vi "XPS_LTA_HS_Jogger.vi"(4 "Axis 2":string="Group7", 5 "Axis 1":string="Group2", 7 "Controller Address":string="192.168.254.254") -> ()   [LabVIEW 2016]
uses:
  <vilib>/Utility/miscctls.llb/LVMinMaxIncTypeDef.ctl
panel:
  in  "Data Entry Limits":T1
  in  "Axis Initial Parameters":T2={"Velocity (units/seconds)"=1.0, "Acceleration (units/seconds²)"=20.0, "Minimum Jerk Time (seconds)"=0.005, "Maximum Jerk Time (seconds)"=0.009} {"Maximum Jerk Time (seconds)" format="%.6e"; "Minimum Jerk Time (seconds)" format="%.6e"; "Acceleration (units/seconds²)" format="%.6e"; "Velocity (units/seconds)" format="%.6e"}
  in  "Mode selector":bool
  in  "Axis 2 Velocity (slow)\nmm/s":dbl=1.0 min=0.0 max=10.0 step=0.0001
  in  "Axis 2 Velocity (fast)\nmm/s":dbl=5.0 min=0.0 max=10.0 step=0.0001
  in  "Velocity (slow)":dbl=1.0 min=0.0 max=5.0 step=0.0001
  in  "Velocity (fast)":dbl=5.0 min=0.0 max=5.0 step=0.0001
  in  "Refresh Time":u32=100 min=50 max=10000 step=1
  in  "Tab Control":enum32{"JOG MODE", "MOVE MODE"}(tab)
  in  "Axis 1 negative":bool
  in  "Axis 1 negative fast":bool
  in  "Axis 1 Positive":bool
  in  "Axis 1 Positive fast":bool
  in  "Axis 2 negative":bool
  in  "Axis 2 negative fast":bool
  in  "Axis 2 Positive":bool
  in  "Axis 2 Positive fast":bool
  in  "Absolute":dbl=5.0 min=0.0 max=50.0
  in  "Absolute Axis 2":dbl=5.0 min=-75.0 max=75.0
  in  "Axis 1 move absolute":bool
  in  "Axis 2 move absolute":bool
  in  "Relative":dbl=1.0 min=-50.0 max=50.0
  in  "Relative Axis 2":dbl=1.0 min=-150.0 max=150.0
  in  "Axis 1 move relative":bool
  in  "Axis 2 move relative":bool
  out "Axis 1 Model":string
  out "Axis 2 Model":string
  in  "stop 2":bool
  out "Axis 2 position":dbl format="%.10f"
  out "Axis 2 Status":string
  out "Axis 1 position":dbl format="%.10f"
  out "Axis 1 Status":string
  in  "Motion parameter":T3={"Velocity (units/s)"=5.0, "Acceleration (units/s²)"=20.0} {"Acceleration (units/s²)" format="%.6f"; "Velocity (units/s)" format="%.6f"}
  in  "stop":bool
  # "Axis 1"
  # "Axis 2"
  # "msec"
  # "Axis 1"
  # "Axis 2"
  # "Axis 1"
  # "Axis 2"
  # "Absolute"
  # "Relative"
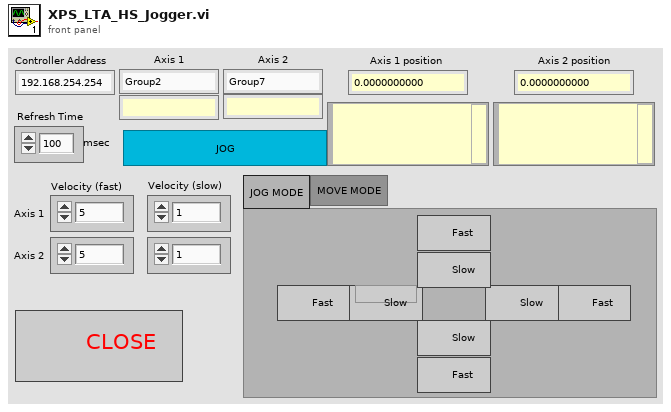
[diagram p1: front panel]
types:
  T1 = typedef "LVMinMaxIncTypeDef.ctl" = cluster{"Minimum":dbl, "Maximum":dbl, "Increment":dbl}
  T2 = cluster{"Velocity (units/seconds)":dbl, "Acceleration (units/seconds²)":dbl, "Minimum Jerk Time (seconds)":dbl, "Maximum Jerk Time (seconds)":dbl}
  T3 = cluster{"Velocity (units/s)":dbl, "Acceleration (units/s²)":dbl}
  T4 = enum32{"Page Enabled", "Page Disabled", "Page Disabled & Grayed"}
  T5 = cluster{"connection TCP":refnum<k5>, "LogTo File":bool, "Log File refnum":refnum<file>, "no error if error log":bool}
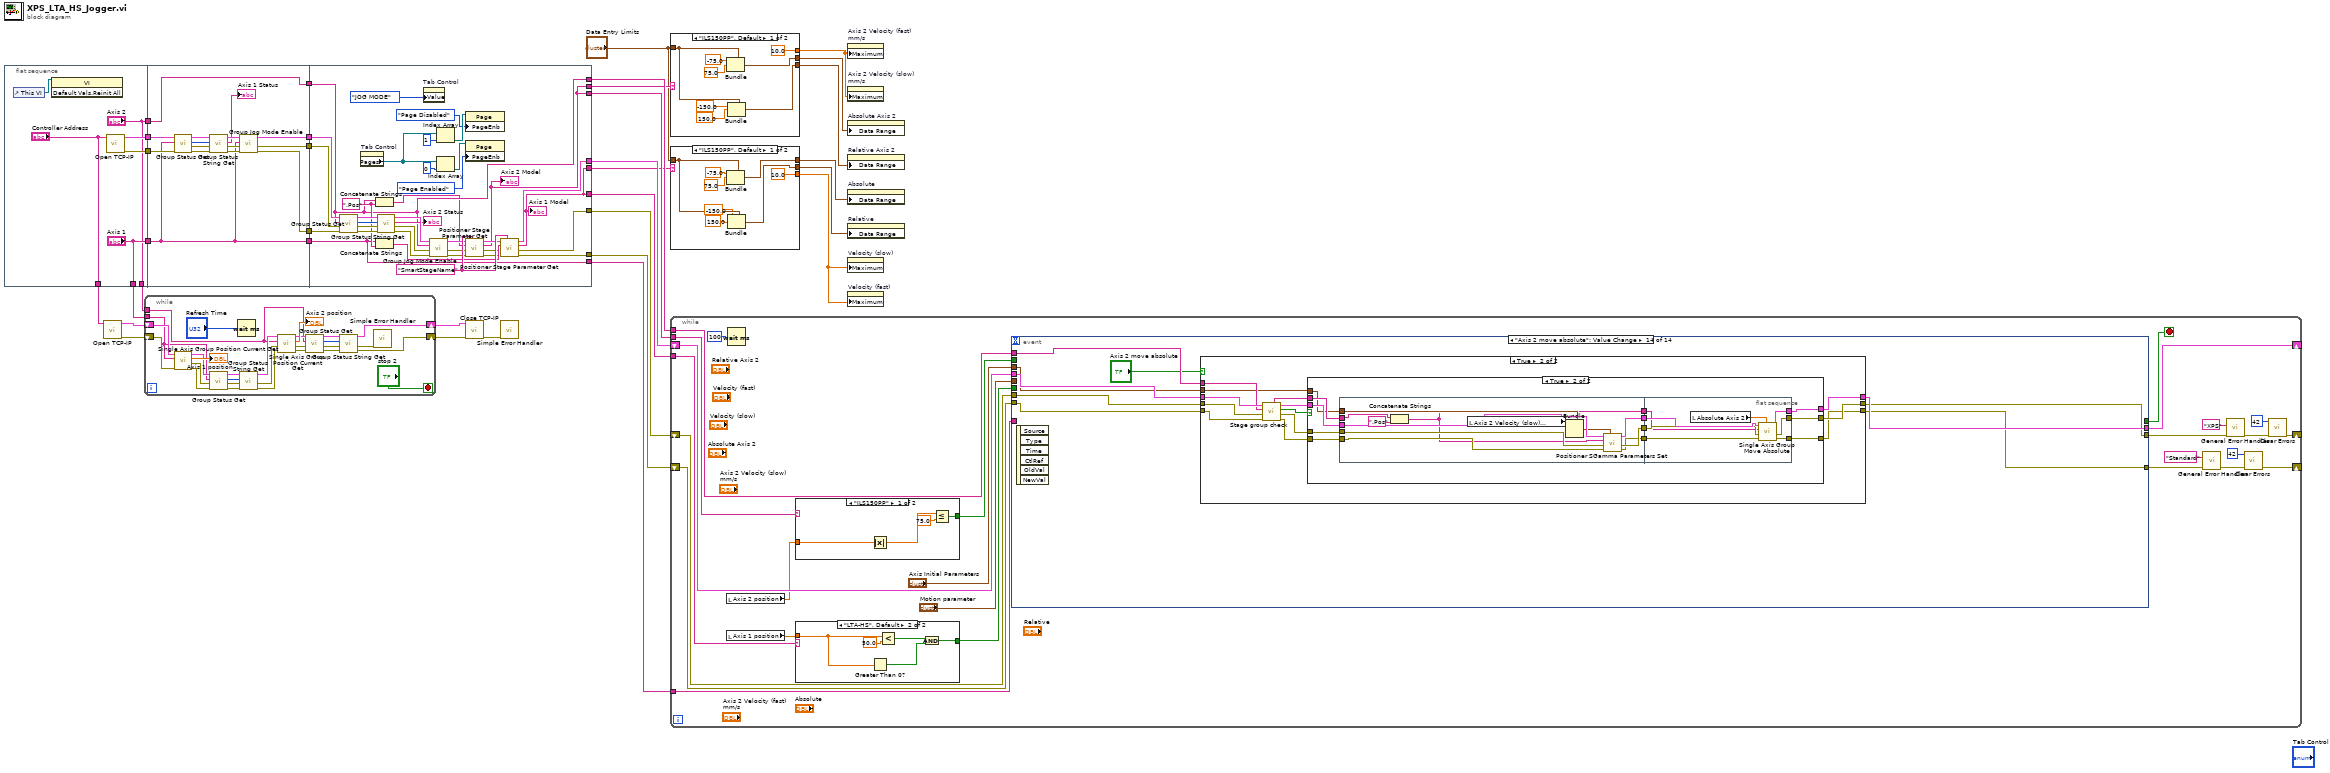
[diagram p0: block diagram]
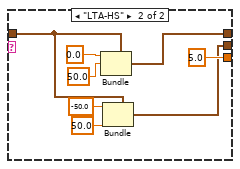
[diagram p2: hidden frame]
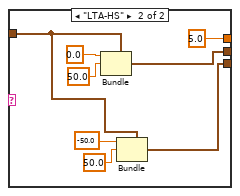
[diagram p3: hidden frame]
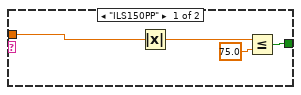
[diagram p4: hidden frame]
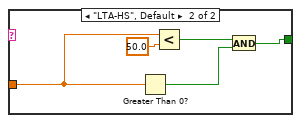
[diagram p5: hidden frame]
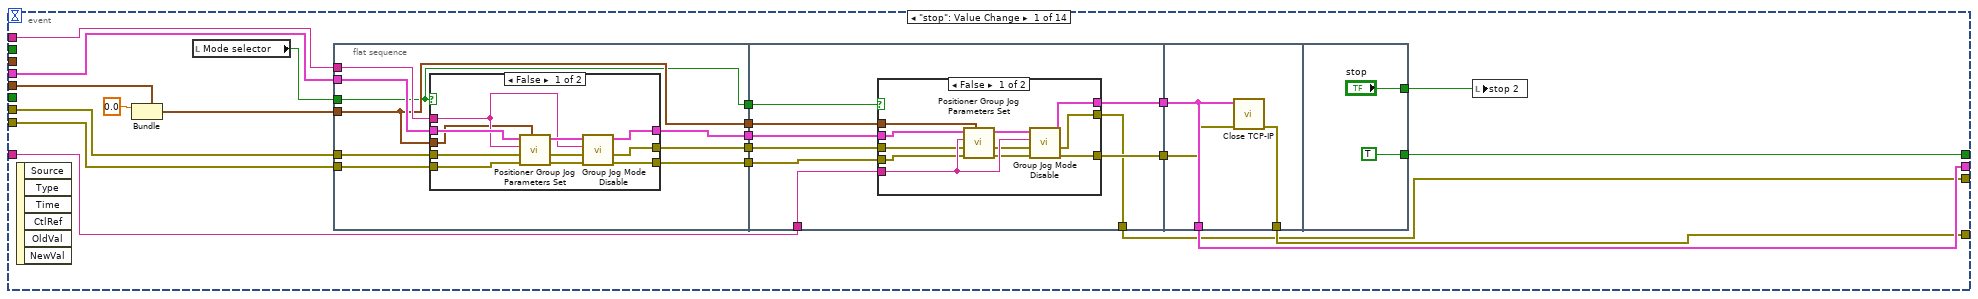
[diagram p6: hidden frame]
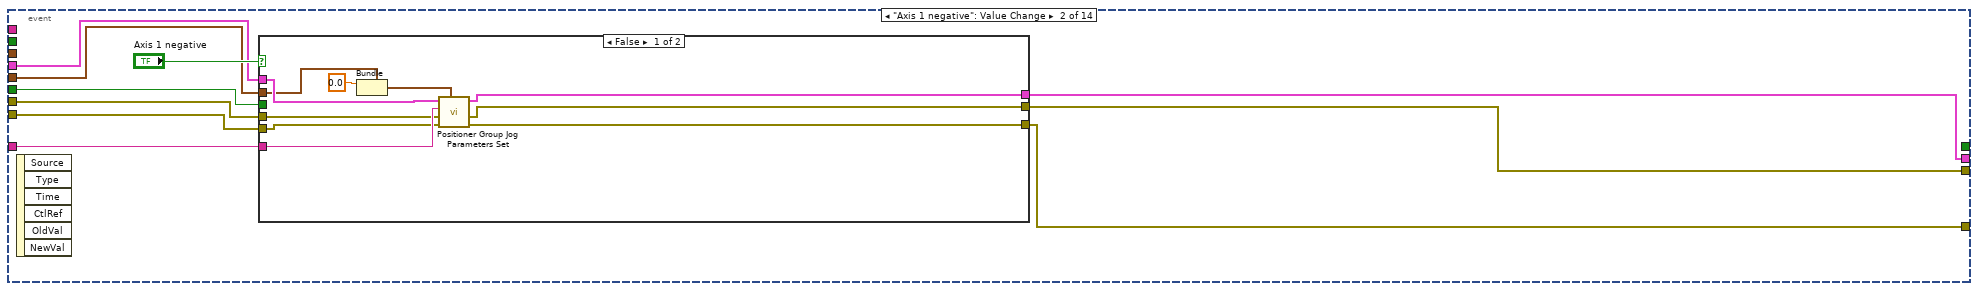
[diagram p9: hidden frame]
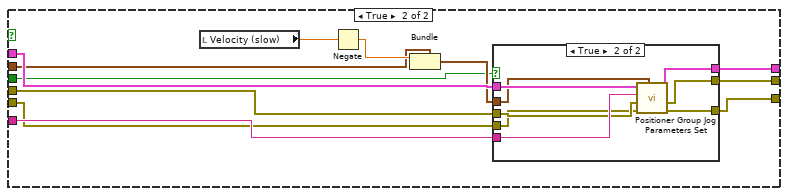
[diagram p10: hidden frame]
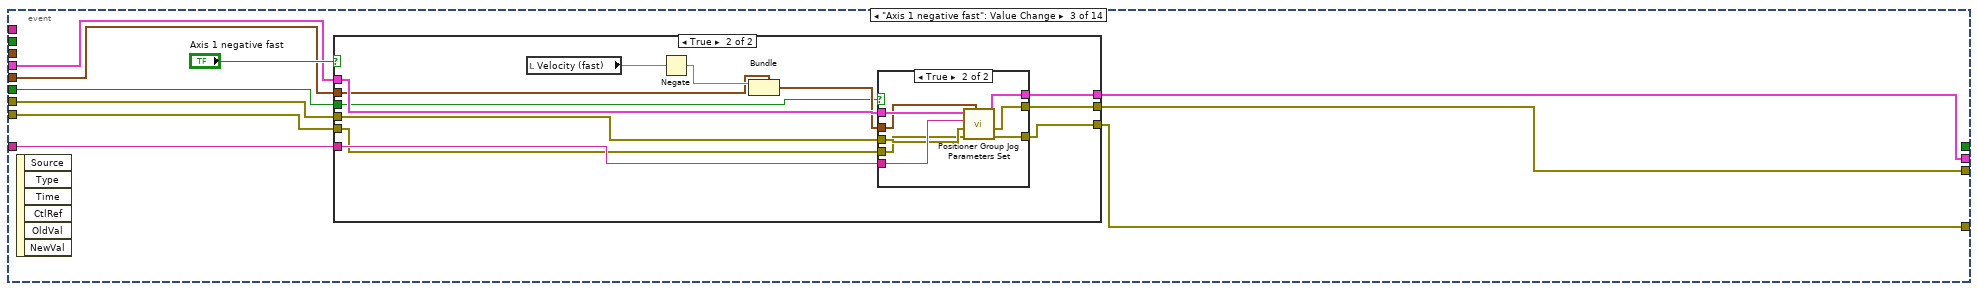
[diagram p12: hidden frame]
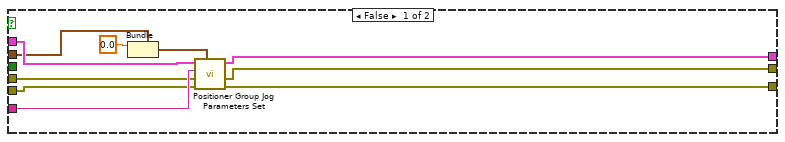
[diagram p13: hidden frame]
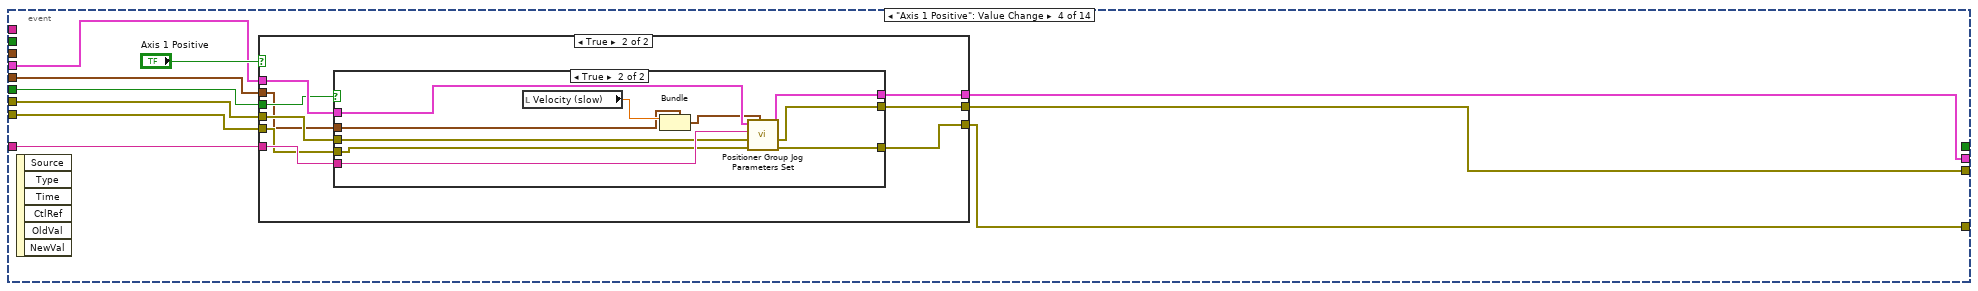
[diagram p15: hidden frame]
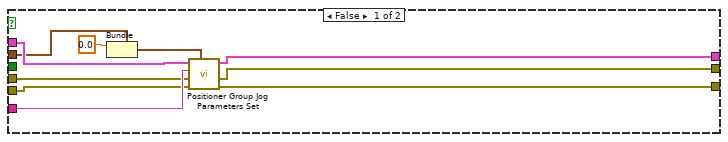
[diagram p16: hidden frame]
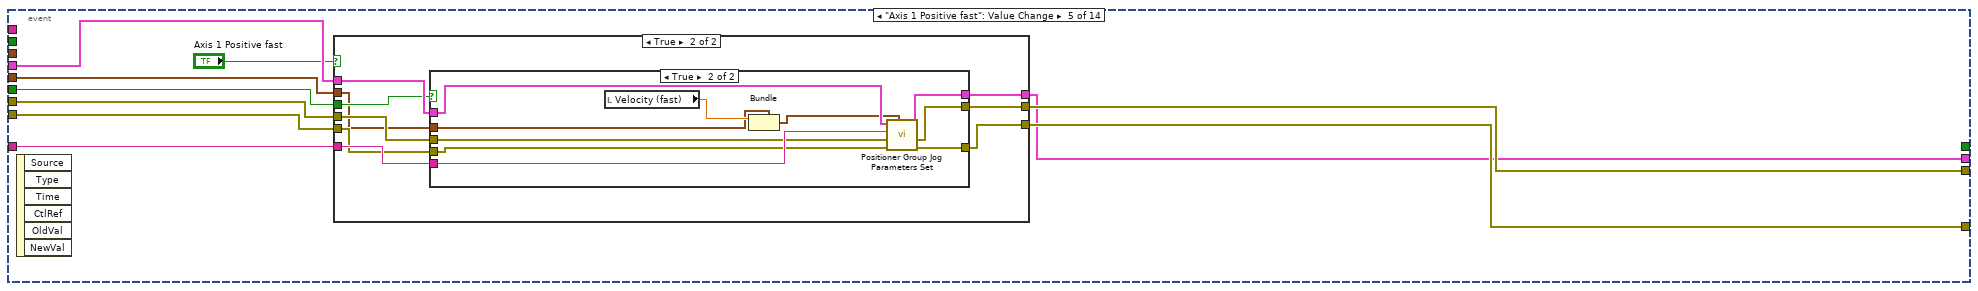
[diagram p18: hidden frame]
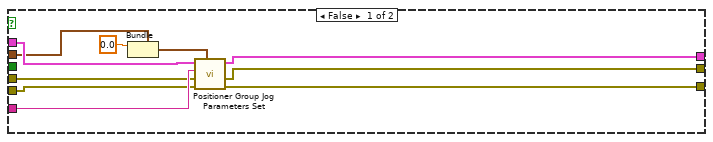
[diagram p19: hidden frame]
diagram:
  n1 = flat-sequence {
    tunnel: ["Axis 1"] -> w30
    tunnel: [w38] -> w29
    tunnel: [w37] -> w28
    tunnel: ["Axis 2"] -> w27
    tunnel: ["Controller Address"] -> w21
    tunnel: ["Axis 1"] -> w16
    tunnel: ["Axis 2"] -> w15
    tunnel: [w54] -> w33
    tunnel: [w53] -> w32
    tunnel: [w52] -> w31
    tunnel: w30 -> [w41]
    tunnel: w29 -> [w47]
    tunnel: w28 -> [w46]
    tunnel: w27 -> [w40]
    tunnel: [w40] -> w26
    tunnel: [w41] -> w24
    tunnel: w33 -> [w87]
    tunnel: w32 -> [w81]
    tunnel: w31 -> [w82]
    tunnel: w26 -> [w73]
    tunnel: w24 -> [w74]
    tunnel: [w65] -> w13
    tunnel: [w76] -> w25
    tunnel: [w74] -> w22
    tunnel: [w73] -> w23
    tunnel: [w68] -> w12
    tunnel: [w63] -> w11
    tunnel: [w64] -> w10
    tunnel: [w64] -> w9
    tunnel: [w63] -> w8
    frame #0 {
      n2 = control-ref of="This VI"() -> (w39:refnum<vi>)
      n3 = invoke class="VI" method="Default Vals.Reinit All"(reference=w39) -> ()  [unwired: 2 in, 3 out]
      n4 = call <userlib>:"Open TCP-IP.vi"("IP address"="Controller Address") -> ("error out"=w38:errorcluster, "Connection ID"=w37:T5)  [unwired: 5 in, 4 out]
    }
    frame #1 {
      n5 = call <userlib>:"Group Status Get.vi"("error in (no error)"=w47, "Group Name (250 c max)"=w41, "connection ID in"=w46) -> ("error out"=w50:errorcluster, "XPS error out"=w51:errorcluster, "Status"=w49:i32, "connection ID out"=w45:T5)  [unwired: 5 in]
      n6 = call <userlib>:"Group Status String Get.vi"("error in (no error)"=w50, "XPS error in (no error)"=w51, "Status #"=w49, "connection ID in"=w45) -> ("error out"=w44:errorcluster, "XPS error out"=w43:errorcluster, "Group Status String"=→"Axis 1 Status":string, "connection ID out"=w48:T5)  [unwired: 4 in]
      n7 = call <userlib>:"Group Jog Mode Enable.vi"("error in (no error)"=w44, "XPS error in (no error)"=w43, "Group Name (250 c max)"=w41, "connection ID in"=w48) -> ("error out"=w52:errorcluster, "XPS error out"=w53:errorcluster, "connection ID out"=w54:T5)  [unwired: 5 in]
    }
    frame #2 {
      w75 = ".Pos" ("string")
      w79 = "SmartStageName" ("Parameter Name (250 c max)")
      n8 = call <userlib>:"Group Status Get.vi"("error in (no error)"=w82, "XPS error in (no error)"=w81, "Group Name (250 c max)"=w73, "connection ID in"=w87) -> ("error out"=w89:errorcluster, "XPS error out"=w90:errorcluster, "Status"=w88:i32, "connection ID out"=w86:T5)  [unwired: 4 in]
      n9 = property on="Tab Control" class="TabCtl (strict)"() -> ("Pages"=w56:refnum<vi>[])  [unwired: 2 in, 2 out]
      n10 = Concatenate Strings(w73, w75) -> (w72:string)
      n11 = Concatenate Strings(w74, w75) -> (w71:string)
      n12 = call <userlib>:"Group Status String Get.vi"("error in (no error)"=w89, "XPS error in (no error)"=w90, "Status #"=w88, "connection ID in"=w86) -> ("error out"=w84:errorcluster, "XPS error out"=w83:errorcluster, "Group Status String"=→"Axis 2 Status":string, "connection ID out"=w85:T5)  [unwired: 4 in]
      n13 = property on="Tab Control" class="TabCtl (strict)"("Value"=enum32{"JOG MODE", "MOVE MODE"}."JOG MODE" ("Tab Control")) -> ()  [unwired: 2 in, 2 out]
      n14 = call <userlib>:"Group Jog Mode Enable.vi"("error in (no error)"=w84, "XPS error in (no error)"=w83, "Group Name (250 c max)"=w73, "connection ID in"=w85) -> ("error out"=w70:errorcluster, "XPS error out"=w67:errorcluster, "connection ID out"=w78:T5)  [unwired: 5 in]
      n15 = Index Array(array=w56, index=1) -> (element=w58:refnum<vi>)
      n16 = Index Array(array=w56, index=0) -> (element=w60:refnum<vi>)
      n17 = property class="Page"(reference=w58, "PageEnb"=T4."Page Disabled" ("Page Enabled State")) -> ()  [unwired: 1 in, 2 out]
      n18 = property class="Page"(reference=w60, "PageEnb"=T4."Page Enabled" ("Page Enabled State")) -> ()  [unwired: 1 in, 2 out]
      n19 = call <userlib>:"Positioner Stage Parameter Get.vi"("Parameter Name (250 c max)"=w79, "error in (no error)"=w70, "XPS error in (no error)"=w67, "Positioner Name (250 c max)"=w72, "connection ID in"=w78) -> ("error out"=w69:errorcluster, "XPS error out"=w66:errorcluster, "Parameter Value"=w64:string, "connection ID out"=w77:T5)  [unwired: 3 in]
      "Axis 2 Model" <- w64
      n20 = call <userlib>:"Positioner Stage Parameter Get.vi"("Parameter Name (250 c max)"=w79, "error in (no error)"=w69, "XPS error in (no error)"=w66, "Positioner Name (250 c max)"=w71, "connection ID in"=w77) -> ("error out"=w68:errorcluster, "XPS error out"=w65:errorcluster, "Parameter Value"=w63:string, "connection ID out"=w76:T5)  [unwired: 3 in]
      "Axis 1 Model" <- w63
    }
  }
  n21 = call <userlib>:"Open TCP-IP.vi"("IP address"=w21) -> ("error out"=w19:errorcluster, "Connection ID"=w20:T5)  [unwired: 5 in, 4 out]
  n22 = while {
    shift-right: [w93] -> w18
    shift-left: w20 -> [w118]
    shift-right: [w92] -> w17
    shift-left: w19 -> [w117]
    tunnel: w16 -> [w109]
    tunnel: w15 -> [w96]
    stop <- "stop 2" stop-if-true
    n23 = call <userlib>:"Single Axis Group Position Current Get.vi"("error in (no error)"=w117, "SingleAxis Group  Name (250 c max)"=w109, "connection ID in"=w118) -> ("error out"=w108:errorcluster, "XPS error out"=w107:errorcluster, "Current Position (units)"=→"Axis 1 position":dbl, "connection ID out"=w112:T5)  [unwired: 5 in]
    n24 = call <userlib>:"Group Status Get.vi"("error in (no error)"=w108, "XPS error in (no error)"=w107, "Group Name (250 c max)"=w109, "connection ID in"=w112) -> ("error out"=w105:errorcluster, "XPS error out"=w106:errorcluster, "Status"=w110:i32, "connection ID out"=w111:T5)  [unwired: 4 in]
    n25 = Wait (ms)(milliseconds to wait="Refresh Time") -> ()  [unwired: 1 out]
    n26 = call <userlib>:"Group Status String Get.vi"("error in (no error)"=w105, "XPS error in (no error)"=w106, "Status #"=w110, "connection ID in"=w111) -> ("error out"=w102:errorcluster, "XPS error out"=w103:errorcluster, "connection ID out"=w104:T5)  [unwired: 4 in, 1 out]
    n27 = call <userlib>:"Single Axis Group Position Current Get.vi"("error in (no error)"=w102, "XPS error in (no error)"=w103, "SingleAxis Group  Name (250 c max)"=w96, "connection ID in"=w104) -> ("error out"=w99:errorcluster, "XPS error out"=w100:errorcluster, "Current Position (units)"=→"Axis 2 position":dbl, "connection ID out"=w101:T5)  [unwired: 4 in]
    n28 = call <userlib>:"Group Status Get.vi"("error in (no error)"=w99, "XPS error in (no error)"=w100, "Group Name (250 c max)"=w96, "connection ID in"=w101) -> ("error out"=w97:errorcluster, "XPS error out"=w98:errorcluster, "Status"=w94:i32, "connection ID out"=w95:T5)  [unwired: 4 in]
    n29 = call <userlib>:"Group Status String Get.vi"("error in (no error)"=w97, "XPS error in (no error)"=w98, "Status #"=w94, "connection ID in"=w95) -> ("error out"=w92:errorcluster, "XPS error out"=w91:errorcluster, "connection ID out"=w93:T5)  [unwired: 4 in, 1 out]
    n30 = call <vilib>:"Simple Error Handler.vi"("error in (no error)"=w91) -> ()  [unwired: 4 in, 5 out]
  }
  n31 = call <userlib>:"Close TCP-IP.vi"("error in (no error)"=w17, "connection ID in"=w18) -> ("Error out"=w14:errorcluster)  [unwired: 9 in]
  n32 = call <vilib>:"Simple Error Handler.vi"("error in (no error)"=w14) -> ()  [unwired: 4 in, 5 out]
  n33 = case shown="\"ILS150PP\", Default" w9 {
    tunnel: [10.0 5.0] -> w7
    tunnel: "Data Entry Limits" -> [w122 w129]
    tunnel: [w123 w131] -> w4
    tunnel: [w120 w127] -> w3
    frame "ILS150PP", Default {
      n34 = Bundle(cluster=w122, "Minimum"=-75.0, "Maximum"=75.0) -> (w123:T1)  [unwired: 1 in]
      n35 = Bundle(cluster=w122, "Minimum"=-150.0, "Maximum"=150.0) -> (w120:T1)  [unwired: 1 in]
    }
    frame "LTA-HS" {
      n36 = Bundle(cluster=w129, "Minimum"=0.0, "Maximum"=50.0) -> (w131:T1)  [unwired: 1 in]
      n37 = Bundle(cluster=w129, "Minimum"=-50.0, "Maximum"=50.0) -> (w127:T1)  [unwired: 1 in]
    }
  }
  n38 = case shown="\"ILS150PP\", Default" w8 {
    tunnel: [10.0 5.0] -> w6
    tunnel: "Data Entry Limits" -> [w139 w146]
    tunnel: [w136 w143] -> w1
    tunnel: [w137 w147] -> w2
    frame "ILS150PP", Default {
      n39 = Bundle(cluster=w139, "Minimum"=-75.0, "Maximum"=75.0) -> (w137:T1)  [unwired: 1 in]
      n40 = Bundle(cluster=w139, "Minimum"=-150.0, "Maximum"=150.0) -> (w136:T1)  [unwired: 1 in]
    }
    frame "LTA-HS" {
      n41 = Bundle(cluster=w146, "Minimum"=0.0, "Maximum"=50.0) -> (w147:T1)  [unwired: 1 in]
      n42 = Bundle(cluster=w146, "Minimum"=-50.0, "Maximum"=50.0) -> (w143:T1)  [unwired: 1 in]
    }
  }
  n43 = while {
    shift-right: [w175] -> _
    shift-left: w25 -> [w176]
    tunnel: w23 -> [w174]
    tunnel: w22 -> [w173]
    shift-right: [w159] -> _
    shift-left: w12 -> [w166]
    shift-right: [w162] -> _
    shift-left: w13 -> [w167]
    tunnel: w11 -> [w154]
    tunnel: w10 -> [w153]
    stop <- w169 stop-if-true
    n44 = local read "Axis 2 position"() -> (w155:dbl)
    n45 = local read "Axis 1 position"() -> (w158:dbl)
    n46 = Wait (ms)(milliseconds to wait=u32 100) -> ()  [unwired: 1 out]
    n47 = case shown="\"ILS150PP\"" w153 {
      tunnel: w155 -> [w187 w192]
      tunnel: [w188 w190] -> w156
      frame "ILS150PP" {
        n48 = Absolute Value(x=w187) -> (abs(x)=w186:dbl)
        n49 = Less Or Equal?(x=w186, y=75.0) -> (x <= y?=w188:bool)
      }
      frame "LTA-HS", Default {
        n50 = Greater Than 0?(x=w192) -> (x > 0?=w191:bool)
        n51 = Less?(x=w192, y=50.0) -> (x < y?=w194:bool)
        n52 = And(x=w194, y=w191) -> (x .and. y?=w190:bool)
      }
    }
    n53 = case shown="\"LTA-HS\", Default" w154 {
      tunnel: w158 -> [w179 w183]
      tunnel: [w177 w181] -> w157
      frame "ILS150PP" {
        n54 = Absolute Value(x=w179) -> (abs(x)=w178:dbl)
        n55 = Less Or Equal?(x=w178, y=75.0) -> (x <= y?=w177:bool)
      }
      frame "LTA-HS", Default {
        n56 = Greater Than 0?(x=w183) -> (x > 0?=w182:bool)
        n57 = Less?(x=w183, y=50.0) -> (x < y?=w185:bool)
        n58 = And(x=w185, y=w182) -> (x .and. y?=w181:bool)
      }
    }
    n59 = event shown="[13] \"Axis 2 move absolute\": Value Change" {
      selector: _ -> [_ _ _ _ _ _ _ _ _ _ _ _ _ _]
      dyn-events: _ -> [_ _ _ _ _ _ _ _ _ _ _ _ _ _]
      timeout: _ -> [_ _ _ _ _ _ _ _ _ _ _ _ _ _]
      tunnel: [w200 w272 w315 w358 w403 w443 w485 w528 w570 w608 w773 w832 w893 w954] -> w170
      tunnel: w176 -> [w215 w275 w318 w361 w404 w445 w488 w531 w573 w615 w779 w839 w900 w962]
      tunnel: [w214 w274 w317 w360 w401 w442 w487 w530 w572 w610 w775 w834 w895 w956] -> w175
      tunnel: [w199 w273 w316 w359 w402 w444 w486 w529 w571 w609 w774 w833 w894 w955] -> w171
      tunnel: w174 -> [w209 _ _ _ _ w441 w484 w527 w569 w611 _ _ w898 w959]
      tunnel: w173 -> [w208 w271 w314 w357 w399 _ _ _ _ w614 w778 w836 _ _]
      tunnel: [w207 _ _ _ _ _ _ _ _ _ _ _ _ _] -> w169
      tunnel: w167 -> [w205 w270 w313 w356 w398 w440 w483 w526 w568 w613 w777 w838 w899 w961]
      tunnel: w166 -> [w201 w269 w312 w355 w397 w439 w482 w525 w567 w612 w776 w837 w897 w960]
      tunnel: w156 -> [_ _ _ _ _ w438 w481 w524 w566 _ _ _ _ _]
      tunnel: w157 -> [_ w268 w311 w354 w396 _ _ _ _ _ _ _ _ _]
      tunnel: "Axis Initial Parameters" -> [_ _ _ _ _ _ _ _ _ _ w772 w840 w901 w958]
      tunnel: "Motion parameter" -> [w198 w267 w310 w353 w395 w437 w480 w523 w565 w607 _ _ _ _]
      event "stop": Value Change {
        n60 = event-data() -> ()  [unwired: 1 in, 6 out]
        n61 = Bundle(cluster=w198, "Velocity (units/s)"=0.0) -> (w210:T3)  [unwired: 1 in]
        n62 = local read "Mode selector"() -> (w196:bool)
        n63 = flat-sequence {
          tunnel: w215 -> [w224]
          tunnel: [w223] -> w212
          tunnel: w210 -> [w217]
          tunnel: w209 -> [w222]
          tunnel: w205 -> [w221]
          tunnel: [w220] -> w204
          tunnel: [w219] -> w202
          tunnel: w201 -> [w218]
          tunnel: [w217] -> w197
          tunnel: w196 -> [w216]
          tunnel: [w216] -> w195
          tunnel: [w246] -> w213
          tunnel: w212 -> [w247]
          tunnel: w208 -> [w245]
          tunnel: w204 -> [w244]
          tunnel: [w243] -> w203
          tunnel: w202 -> [w242]
          tunnel: [w241] -> w199
          tunnel: w197 -> [w240]
          tunnel: w195 -> [w239]
          tunnel: [w264] -> w214
          tunnel: w213 -> [w264]
          tunnel: w203 -> [w263]
          tunnel: [w262] -> w200
          tunnel: [TRUE] -> w207
          tunnel: ["stop"] -> w206
          frame #0 {
            n64 = case shown="False" w216 {
              tunnel: w224 -> [w234 w238]
              tunnel: [w233 w238] -> w223
              tunnel: w222 -> [w232 _]
              tunnel: w221 -> [w231 w237]
              tunnel: [w229 w237] -> w220
              tunnel: [w228 w236] -> w219
              tunnel: w218 -> [w226 w236]
              tunnel: w217 -> [w225 _]
              frame False {
                n65 = call <userlib>:"Positioner Group Jog Parameters Set.vi"("Group Jog parameters"=w225, "error in (no error)"=w226, "XPS error in (no error)"=w231, "Positioner Name (250 c max)"=w232, "connection ID in"=w234) -> ("error out"=w227:errorcluster, "XPS error out"=w230:errorcluster, "connection ID out"=w235:T5)  [unwired: 4 in]
                n66 = call <userlib>:"Group Jog Mode Disable.vi"("error in (no error)"=w227, "XPS error in (no error)"=w230, "Group Name (250 c max)"=w232, "connection ID in"=w235) -> ("error out"=w228:errorcluster, "XPS error out"=w229:errorcluster, "connection ID out"=w233:T5)  [unwired: 5 in]
              }
              frame True {
              }
            }
          }
          frame #1 {
            n67 = case shown="False" w239 {
              tunnel: w247 -> [w258 w261]
              tunnel: [w256 w261] -> w246
              tunnel: w245 -> [w255 _]
              tunnel: w244 -> [w254 w260]
              tunnel: [w252 w259] -> w243
              tunnel: w242 -> [w250 w259]
              tunnel: [w249 w260] -> w241
              tunnel: w240 -> [w248 _]
              frame False {
                n68 = call <userlib>:"Positioner Group Jog Parameters Set.vi"("Group Jog parameters"=w248, "error in (no error)"=w250, "XPS error in (no error)"=w254, "Positioner Name (250 c max)"=w255, "connection ID in"=w258) -> ("error out"=w251:errorcluster, "XPS error out"=w253:errorcluster, "connection ID out"=w257:T5)  [unwired: 4 in]
                n69 = call <userlib>:"Group Jog Mode Disable.vi"("error in (no error)"=w251, "XPS error in (no error)"=w253, "Group Name (250 c max)"=w255, "connection ID in"=w257) -> ("error out"=w252:errorcluster, "XPS error out"=w249:errorcluster, "connection ID out"=w256:T5)  [unwired: 5 in]
              }
              frame True {
              }
            }
          }
          frame #2 {
            n70 = call <userlib>:"Close TCP-IP.vi"("error in (no error)"=w263, "connection ID in"=w264) -> ("Error out"=w262:errorcluster)  [unwired: 9 in]
          }
          frame #3 {
          }
        }
        n71 = local write "stop 2"(w206) -> ()
      }
      event "Axis 1 negative": Value Change {
        n72 = event-data() -> ()  [unwired: 1 in, 6 out]
        n73 = case shown="False" "Axis 1 negative" {
          tunnel: w275 -> [w286 w298]
          tunnel: [w285 w297] -> w274
          tunnel: [w284 w296] -> w273
          tunnel: [w283 w295] -> w272
          tunnel: w271 -> [w282 w294]
          tunnel: w270 -> [w280 w292]
          tunnel: w269 -> [w279 w291]
          tunnel: w268 -> [_ w290]
          tunnel: w267 -> [w278 w287]
          frame False {
            n74 = Bundle(cluster=w278, "Velocity (units/s)"=0.0) -> (w277:T3)  [unwired: 1 in]
            n75 = call <userlib>:"Positioner Group Jog Parameters Set.vi"("Group Jog parameters"=w277, "error in (no error)"=w279, "XPS error in (no error)"=w280, "Positioner Name (250 c max)"=w282, "connection ID in"=w286) -> ("error out"=w283:errorcluster, "XPS error out"=w284:errorcluster, "connection ID out"=w285:T5)  [unwired: 4 in]
          }
          frame True {
            n76 = local read "Velocity (slow)"() -> (w289:dbl)
            n77 = Negate(x=w289) -> (-x=w288:dbl)
            n78 = Bundle(cluster=w287, "Velocity (units/s)"=w288) -> (w293:T3)  [unwired: 1 in]
            n79 = case shown="True" w290 {
              tunnel: w298 -> [w301 w309]
              tunnel: [w301 w308] -> w297
              tunnel: [w300 w307] -> w296
              tunnel: [w299 w306] -> w295
              tunnel: w294 -> [_ w305]
              tunnel: w293 -> [_ w304]
              tunnel: w292 -> [w300 w303]
              tunnel: w291 -> [w299 w302]
              frame False {
              }
              frame True {
                n80 = call <userlib>:"Positioner Group Jog Parameters Set.vi"("Group Jog parameters"=w304, "error in (no error)"=w302, "XPS error in (no error)"=w303, "Positioner Name (250 c max)"=w305, "connection ID in"=w309) -> ("error out"=w306:errorcluster, "XPS error out"=w307:errorcluster, "connection ID out"=w308:T5)  [unwired: 4 in]
              }
            }
          }
        }
      }
      event "Axis 1 negative fast": Value Change {
        n81 = event-data() -> ()  [unwired: 1 in, 6 out]
        n82 = case shown="True" "Axis 1 negative fast" {
          tunnel: w318 -> [w329 w341]
          tunnel: [w328 w340] -> w317
          tunnel: [w327 w339] -> w316
          tunnel: [w326 w338] -> w315
          tunnel: w314 -> [w325 w337]
          tunnel: w313 -> [w323 w334]
          tunnel: w312 -> [w322 w333]
          tunnel: w311 -> [_ w332]
          tunnel: w310 -> [w321 w330]
          frame False {
            n83 = Bundle(cluster=w321, "Velocity (units/s)"=0.0) -> (w320:T3)  [unwired: 1 in]
            n84 = call <userlib>:"Positioner Group Jog Parameters Set.vi"("Group Jog parameters"=w320, "error in (no error)"=w322, "XPS error in (no error)"=w323, "Positioner Name (250 c max)"=w325, "connection ID in"=w329) -> ("error out"=w326:errorcluster, "XPS error out"=w327:errorcluster, "connection ID out"=w328:T5)  [unwired: 4 in]
          }
          frame True {
            n85 = local read "Velocity (fast)"() -> (w331:dbl)
            n86 = Negate(x=w331) -> (-x=w336:dbl)
            n87 = Bundle(cluster=w330, "Velocity (units/s)"=w336) -> (w335:T3)  [unwired: 1 in]
            n88 = case shown="True" w332 {
              tunnel: w341 -> [w342 w352]
              tunnel: [w342 w351] -> w340
              tunnel: [w343 w350] -> w339
              tunnel: [w344 w349] -> w338
              tunnel: w337 -> [_ w348]
              tunnel: w335 -> [_ w347]
              tunnel: w334 -> [w343 w346]
              tunnel: w333 -> [w344 w345]
              frame False {
              }
              frame True {
                n89 = call <userlib>:"Positioner Group Jog Parameters Set.vi"("Group Jog parameters"=w347, "error in (no error)"=w345, "XPS error in (no error)"=w346, "Positioner Name (250 c max)"=w348, "connection ID in"=w352) -> ("error out"=w349:errorcluster, "XPS error out"=w350:errorcluster, "connection ID out"=w351:T5)  [unwired: 4 in]
              }
            }
          }
        }
      }
      event "Axis 1 Positive": Value Change {
        n90 = event-data() -> ()  [unwired: 1 in, 6 out]
        n91 = case shown="True" "Axis 1 Positive" {
          tunnel: w361 -> [w372 w381]
          tunnel: [w371 w380] -> w360
          tunnel: [w370 w379] -> w359
          tunnel: [w369 w378] -> w358
          tunnel: w357 -> [w368 w377]
          tunnel: w356 -> [w366 w376]
          tunnel: w355 -> [w365 w375]
          tunnel: w354 -> [_ w374]
          tunnel: w353 -> [w364 w373]
          frame False {
            n92 = Bundle(cluster=w364, "Velocity (units/s)"=0.0) -> (w363:T3)  [unwired: 1 in]
            n93 = call <userlib>:"Positioner Group Jog Parameters Set.vi"("Group Jog parameters"=w363, "error in (no error)"=w365, "XPS error in (no error)"=w366, "Positioner Name (250 c max)"=w368, "connection ID in"=w372) -> ("error out"=w369:errorcluster, "XPS error out"=w370:errorcluster, "connection ID out"=w371:T5)  [unwired: 4 in]
          }
          frame True {
            n94 = case shown="True" w374 {
              tunnel: w381 -> [w382 w394]
              tunnel: [w382 w393] -> w380
              tunnel: [w384 w392] -> w379
              tunnel: [w383 w391] -> w378
              tunnel: w377 -> [_ w390]
              tunnel: w376 -> [w384 w389]
              tunnel: w375 -> [w383 w388]
              tunnel: w373 -> [_ w385]
              frame False {
              }
              frame True {
                n95 = local read "Velocity (slow)"() -> (w387:dbl)
                n96 = Bundle(cluster=w385, "Velocity (units/s)"=w387) -> (w386:T3)  [unwired: 1 in]
                n97 = call <userlib>:"Positioner Group Jog Parameters Set.vi"("Group Jog parameters"=w386, "error in (no error)"=w388, "XPS error in (no error)"=w389, "Positioner Name (250 c max)"=w390, "connection ID in"=w394) -> ("error out"=w391:errorcluster, "XPS error out"=w392:errorcluster, "connection ID out"=w393:T5)  [unwired: 4 in]
              }
            }
          }
        }
      }
      event "Axis 1 Positive fast": Value Change {
        n98 = event-data() -> ()  [unwired: 1 in, 6 out]
        n99 = case shown="True" "Axis 1 Positive fast" {
          tunnel: w404 -> [w414 w423]
          tunnel: [w411 w420] -> w403
          tunnel: [w412 w421] -> w402
          tunnel: [w413 w422] -> w401
          tunnel: w399 -> [w410 w419]
          tunnel: w398 -> [w408 w417]
          tunnel: w397 -> [w407 w418]
          tunnel: w396 -> [_ w416]
          tunnel: w395 -> [w406 w415]
          frame False {
            n100 = Bundle(cluster=w406, "Velocity (units/s)"=0.0) -> (w405:T3)  [unwired: 1 in]
            n101 = call <userlib>:"Positioner Group Jog Parameters Set.vi"("Group Jog parameters"=w405, "error in (no error)"=w407, "XPS error in (no error)"=w408, "Positioner Name (250 c max)"=w410, "connection ID in"=w414) -> ("error out"=w411:errorcluster, "XPS error out"=w412:errorcluster, "connection ID out"=w413:T5)  [unwired: 4 in]
          }
          frame True {
            n102 = case shown="True" w416 {
              tunnel: w423 -> [w424 w436]
              tunnel: [w424 w435] -> w422
              tunnel: [w426 w434] -> w421
              tunnel: [w425 w433] -> w420
              tunnel: w419 -> [_ w432]
              tunnel: w418 -> [w425 w431]
              tunnel: w417 -> [w426 w430]
              tunnel: w415 -> [_ w427]
              frame False {
              }
              frame True {
                n103 = local read "Velocity (fast)"() -> (w428:dbl)
                n104 = Bundle(cluster=w427, "Velocity (units/s)"=w428) -> (w429:T3)  [unwired: 1 in]
                n105 = call <userlib>:"Positioner Group Jog Parameters Set.vi"("Group Jog parameters"=w429, "error in (no error)"=w431, "XPS error in (no error)"=w430, "Positioner Name (250 c max)"=w432, "connection ID in"=w436) -> ("error out"=w433:errorcluster, "XPS error out"=w434:errorcluster, "connection ID out"=w435:T5)  [unwired: 4 in]
              }
            }
          }
        }
      }
      event "Axis 2 negative": Value Change {
        n106 = event-data() -> ()  [unwired: 1 in, 6 out]
        n107 = case shown="True" "Axis 2 negative" {
          tunnel: w445 -> [w456 w468]
          tunnel: [w454 w466] -> w444
          tunnel: [w453 w465] -> w443
          tunnel: [w455 w467] -> w442
          tunnel: w441 -> [w452 w464]
          tunnel: w440 -> [w450 w461]
          tunnel: w439 -> [w449 w460]
          tunnel: w438 -> [_ w459]
          tunnel: w437 -> [w448 w457]
          frame False {
            n108 = Bundle(cluster=w448, "Velocity (units/s)"=0.0) -> (w447:T3)  [unwired: 1 in]
            n109 = call <userlib>:"Positioner Group Jog Parameters Set.vi"("Group Jog parameters"=w447, "error in (no error)"=w449, "XPS error in (no error)"=w450, "Positioner Name (250 c max)"=w452, "connection ID in"=w456) -> ("error out"=w453:errorcluster, "XPS error out"=w454:errorcluster, "connection ID out"=w455:T5)  [unwired: 4 in]
          }
          frame True {
            n110 = local read "Axis 2 Velocity (slow)\nmm/s"() -> (w458:dbl)
            n111 = Negate(x=w458) -> (-x=w463:dbl)
            n112 = Bundle(cluster=w457, "Velocity (units/s)"=w463) -> (w462:T3)  [unwired: 1 in]
            n113 = case shown="True" w459 {
              tunnel: w468 -> [w471 w479]
              tunnel: [w471 w478] -> w467
              tunnel: [w470 w477] -> w466
              tunnel: [w469 w476] -> w465
              tunnel: w464 -> [_ w475]
              tunnel: w462 -> [_ w474]
              tunnel: w461 -> [w470 w473]
              tunnel: w460 -> [w469 w472]
              frame False {
              }
              frame True {
                n114 = call <userlib>:"Positioner Group Jog Parameters Set.vi"("Group Jog parameters"=w474, "error in (no error)"=w472, "XPS error in (no error)"=w473, "Positioner Name (250 c max)"=w475, "connection ID in"=w479) -> ("error out"=w476:errorcluster, "XPS error out"=w477:errorcluster, "connection ID out"=w478:T5)  [unwired: 4 in]
              }
            }
          }
        }
      }
      event "Axis 2 negative fast": Value Change {
        n115 = event-data() -> ()  [unwired: 1 in, 6 out]
        n116 = case shown="True" "Axis 2 negative fast" {
          tunnel: w488 -> [w499 w511]
          tunnel: [w498 w510] -> w487
          tunnel: [w497 w509] -> w486
          tunnel: [w496 w508] -> w485
          tunnel: w484 -> [w495 w507]
          tunnel: w483 -> [w493 w504]
          tunnel: w482 -> [w492 w503]
          tunnel: w481 -> [_ w502]
          tunnel: w480 -> [w491 w500]
          frame False {
            n117 = Bundle(cluster=w491, "Velocity (units/s)"=0.0) -> (w490:T3)  [unwired: 1 in]
            n118 = call <userlib>:"Positioner Group Jog Parameters Set.vi"("Group Jog parameters"=w490, "error in (no error)"=w492, "XPS error in (no error)"=w493, "Positioner Name (250 c max)"=w495, "connection ID in"=w499) -> ("error out"=w496:errorcluster, "XPS error out"=w497:errorcluster, "connection ID out"=w498:T5)  [unwired: 4 in]
          }
          frame True {
            n119 = local read "Axis 2 Velocity (fast)\nmm/s"() -> (w501:dbl)
            n120 = Negate(x=w501) -> (-x=w506:dbl)
            n121 = Bundle(cluster=w500, "Velocity (units/s)"=w506) -> (w505:T3)  [unwired: 1 in]
            n122 = case shown="True" w502 {
              tunnel: w511 -> [w514 w522]
              tunnel: [w514 w521] -> w510
              tunnel: [w513 w520] -> w509
              tunnel: [w512 w519] -> w508
              tunnel: w507 -> [_ w518]
              tunnel: w505 -> [_ w517]
              tunnel: w504 -> [w513 w516]
              tunnel: w503 -> [w512 w515]
              frame False {
              }
              frame True {
                n123 = call <userlib>:"Positioner Group Jog Parameters Set.vi"("Group Jog parameters"=w517, "error in (no error)"=w515, "XPS error in (no error)"=w516, "Positioner Name (250 c max)"=w518, "connection ID in"=w522) -> ("error out"=w519:errorcluster, "XPS error out"=w520:errorcluster, "connection ID out"=w521:T5)  [unwired: 4 in]
              }
            }
          }
        }
      }
      event "Axis 2 Positive": Value Change {
        n124 = event-data() -> ()  [unwired: 1 in, 6 out]
        n125 = case shown="True" "Axis 2 Positive" {
          tunnel: w531 -> [w542 w551]
          tunnel: [w541 w550] -> w530
          tunnel: [w540 w549] -> w529
          tunnel: [w539 w548] -> w528
          tunnel: w527 -> [w538 w547]
          tunnel: w526 -> [w535 w546]
          tunnel: w525 -> [w536 w545]
          tunnel: w524 -> [_ w544]
          tunnel: w523 -> [w534 w543]
          frame False {
            n126 = Bundle(cluster=w534, "Velocity (units/s)"=0.0) -> (w533:T3)  [unwired: 1 in]
            n127 = call <userlib>:"Positioner Group Jog Parameters Set.vi"("Group Jog parameters"=w533, "error in (no error)"=w536, "XPS error in (no error)"=w535, "Positioner Name (250 c max)"=w538, "connection ID in"=w542) -> ("error out"=w539:errorcluster, "XPS error out"=w540:errorcluster, "connection ID out"=w541:T5)  [unwired: 4 in]
          }
          frame True {
            n128 = case shown="True" w544 {
              tunnel: w551 -> [w554 w564]
              tunnel: [w554 w563] -> w550
              tunnel: [w553 w562] -> w549
              tunnel: [w552 w561] -> w548
              tunnel: w547 -> [_ w560]
              tunnel: w546 -> [w553 w559]
              tunnel: w545 -> [w552 w558]
              tunnel: w543 -> [_ w555]
              frame False {
              }
              frame True {
                n129 = local read "Axis 2 Velocity (slow)\nmm/s"() -> (w556:dbl)
                n130 = Bundle(cluster=w555, "Velocity (units/s)"=w556) -> (w557:T3)  [unwired: 1 in]
                n131 = call <userlib>:"Positioner Group Jog Parameters Set.vi"("Group Jog parameters"=w557, "error in (no error)"=w558, "XPS error in (no error)"=w559, "Positioner Name (250 c max)"=w560, "connection ID in"=w564) -> ("error out"=w561:errorcluster, "XPS error out"=w562:errorcluster, "connection ID out"=w563:T5)  [unwired: 4 in]
              }
            }
          }
        }
      }
      event "Axis 2 Positive fast": Value Change {
        n132 = event-data() -> ()  [unwired: 1 in, 6 out]
        n133 = case shown="True" "Axis 2 Positive fast" {
          tunnel: w573 -> [w584 w593]
          tunnel: [w583 w590] -> w572
          tunnel: [w582 w591] -> w571
          tunnel: [w581 w592] -> w570
          tunnel: w569 -> [w580 w589]
          tunnel: w568 -> [w577 w588]
          tunnel: w567 -> [w578 w587]
          tunnel: w566 -> [_ w586]
          tunnel: w565 -> [w576 w585]
          frame False {
            n134 = Bundle(cluster=w576, "Velocity (units/s)"=0.0) -> (w575:T3)  [unwired: 1 in]
            n135 = call <userlib>:"Positioner Group Jog Parameters Set.vi"("Group Jog parameters"=w575, "error in (no error)"=w578, "XPS error in (no error)"=w577, "Positioner Name (250 c max)"=w580, "connection ID in"=w584) -> ("error out"=w581:errorcluster, "XPS error out"=w582:errorcluster, "connection ID out"=w583:T5)  [unwired: 4 in]
          }
          frame True {
            n136 = case shown="True" w586 {
              tunnel: w593 -> [w596 w606]
              tunnel: [w594 w605] -> w592
              tunnel: [w595 w604] -> w591
              tunnel: [w596 w603] -> w590
              tunnel: w589 -> [_ w602]
              tunnel: w588 -> [w595 w601]
              tunnel: w587 -> [w594 w600]
              tunnel: w585 -> [_ w597]
              frame False {
              }
              frame True {
                n137 = local read "Axis 2 Velocity (fast)\nmm/s"() -> (w598:dbl)
                n138 = Bundle(cluster=w597, "Velocity (units/s)"=w598) -> (w599:T3)  [unwired: 1 in]
                n139 = call <userlib>:"Positioner Group Jog Parameters Set.vi"("Group Jog parameters"=w599, "error in (no error)"=w600, "XPS error in (no error)"=w601, "Positioner Name (250 c max)"=w602, "connection ID in"=w606) -> ("error out"=w605:errorcluster, "XPS error out"=w604:errorcluster, "connection ID out"=w603:T5)  [unwired: 4 in]
              }
            }
          }
        }
      }
      event "Mode selector": Value Change {
        n140 = event-data() -> ()  [unwired: 1 in, 6 out]
        n141 = case shown="False" "Mode selector" {
          tunnel: w615 -> [w631 w701]
          tunnel: w614 -> [w627 w699]
          tunnel: w613 -> [w630 w697]
          tunnel: w612 -> [w629 w696]
          tunnel: w611 -> [w628 w698]
          tunnel: [w634 w712] -> w610
          tunnel: [w633 w711] -> w609
          tunnel: [w632 w710] -> w608
          tunnel: w607 -> [_ w695]
          frame False {
            n142 = call "Stage group check.vi"("error in (no error)"=w629, "XPS error in (no error)"=w630, "Group Name (250 c max)"=w627, "connection ID in"=w631) -> ("error out"=w619:errorcluster, "XPS error out"=w620:errorcluster, "Stages ready?"=w617:bool, "connection ID out"=w624:T5, "Group Name (250 c max) 2"=w626:string)  [unwired: 3 in]
            n143 = call "Stage group check.vi"("error in (no error)"=w619, "XPS error in (no error)"=w620, "Group Name (250 c max)"=w628, "connection ID in"=w624) -> ("error out"=w621:errorcluster, "XPS error out"=w622:errorcluster, "Stages ready?"=w618:bool, "connection ID out"=w623:T5, "Group Name (250 c max) 2"=w625:string)  [unwired: 3 in]
            n144 = And(x=w617, y=w618) -> (x .and. y?=w635:bool)
            n145 = case shown="True" w635 {
              tunnel: [w636 w651] -> w634
              tunnel: [w637 w650] -> w633
              tunnel: [w638 w649] -> w632
              tunnel: w625 -> [_ w647]
              tunnel: w626 -> [_ w646]
              tunnel: w623 -> [w636 w645]
              tunnel: w622 -> [w637 w644]
              tunnel: w621 -> [w638 w643]
              frame False {
                n146 = One Button Dialog(message="Axes are not ready") -> ()  [unwired: 1 in, 1 out]
              }
              frame True {
                n147 = flat-sequence {
                  tunnel: [w660] -> w653
                  tunnel: [w659] -> w652
                  tunnel: [w658] -> w648
                  tunnel: w646 -> [w657]
                  tunnel: w645 -> [w656]
                  tunnel: w644 -> [w655]
                  tunnel: w643 -> [w654]
                  tunnel: w653 -> [w675]
                  tunnel: w652 -> [w674]
                  tunnel: w648 -> [w670]
                  tunnel: w647 -> [w669]
                  tunnel: [w673] -> w642
                  tunnel: [w672] -> w641
                  tunnel: [w671] -> w640
                  tunnel: [w692] -> w649
                  tunnel: [w693] -> w650
                  tunnel: [w694] -> w651
                  tunnel: w642 -> [w694]
                  tunnel: w641 -> [w693]
                  tunnel: w640 -> [w692]
                  frame #0 {
                    n148 = call <userlib>:"Group Status Get.vi"("error in (no error)"=w654, "XPS error in (no error)"=w655, "Group Name (250 c max)"=w657, "connection ID in"=w656) -> ("error out"=w667:errorcluster, "XPS error out"=w668:errorcluster, "Status"=w666:i32, "connection ID out"=w664:T5)  [unwired: 4 in]
                    n149 = call <userlib>:"Group Status String Get.vi"("error in (no error)"=w667, "XPS error in (no error)"=w668, "Status #"=w666, "connection ID in"=w664) -> ("error out"=w663:errorcluster, "XPS error out"=w662:errorcluster, "Group Status String"=w661:string, "connection ID out"=w665:T5)  [unwired: 4 in]
                    n150 = local write "Axis 1 Status"(w661) -> ()
                    n151 = call <userlib>:"Group Jog Mode Enable.vi"("error in (no error)"=w663, "XPS error in (no error)"=w662, "Group Name (250 c max)"=w657, "connection ID in"=w665) -> ("error out"=w660:errorcluster, "XPS error out"=w659:errorcluster, "connection ID out"=w658:T5)  [unwired: 5 in]
                  }
                  frame #1 {
                    n152 = call <userlib>:"Group Status Get.vi"("error in (no error)"=w675, "XPS error in (no error)"=w674, "Group Name (250 c max)"=w669, "connection ID in"=w670) -> ("error out"=w682:errorcluster, "XPS error out"=w683:errorcluster, "Status"=w681:i32, "connection ID out"=w679:T5)  [unwired: 4 in]
                    n153 = call <userlib>:"Group Status String Get.vi"("error in (no error)"=w682, "XPS error in (no error)"=w683, "Status #"=w681, "connection ID in"=w679) -> ("error out"=w678:errorcluster, "XPS error out"=w677:errorcluster, "Group Status String"=w676:string, "connection ID out"=w680:T5)  [unwired: 4 in]
                    n154 = local write "Axis 2 Status"(w676) -> ()
                    n155 = call <userlib>:"Group Jog Mode Enable.vi"("error in (no error)"=w678, "XPS error in (no error)"=w677, "Group Name (250 c max)"=w669, "connection ID in"=w680) -> ("error out"=w671:errorcluster, "XPS error out"=w672:errorcluster, "connection ID out"=w673:T5)  [unwired: 5 in]
                  }
                  frame #2 {
                    n156 = property on="Tab Control" class="TabCtl (strict)"() -> ("Pages"=w685:refnum<vi>[])  [unwired: 2 in, 2 out]
                    n157 = property on="Tab Control" class="TabCtl (strict)"("Value"=enum32{"JOG MODE", "MOVE MODE"}."JOG MODE" ("Tab Control")) -> ()  [unwired: 2 in, 2 out]
                    n158 = Index Array(array=w685, index=1) -> (element=w687:refnum<vi>)
                    n159 = Index Array(array=w685, index=0) -> (element=w689:refnum<vi>)
                    n160 = property class="Page"(reference=w687, "PageEnb"=T4."Page Disabled" ("Page Enabled State")) -> ()  [unwired: 1 in, 2 out]
                    n161 = property class="Page"(reference=w689, "PageEnb"=T4."Page Enabled" ("Page Enabled State")) -> ()  [unwired: 1 in, 2 out]
                  }
                }
              }
            }
          }
          frame True {
            w704 = 44
            n162 = call <userlib>:"Group Status Get.vi"("error in (no error)"=w696, "XPS error in (no error)"=w697, "Group Name (250 c max)"=w698, "connection ID in"=w701) -> ("error out"=w708:errorcluster, "XPS error out"=w707:errorcluster, "Status"=w705:i32, "connection ID out"=w709:T5)  [unwired: 4 in]
            n163 = call <userlib>:"Group Status Get.vi"("error in (no error)"=w708, "XPS error in (no error)"=w707, "Group Name (250 c max)"=w699, "connection ID in"=w709) -> ("error out"=w702:errorcluster, "XPS error out"=w703:errorcluster, "Status"=w706:i32, "connection ID out"=w700:T5)  [unwired: 4 in]
            n164 = Equal?(x=w705, y=w704) -> (x = y?=w714:bool)
            n165 = Equal?(x=w706, y=w704) -> (x = y?=w715:bool)
            n166 = And(x=w715, y=w714) -> (x .and. y?=w713:bool)
            n167 = case shown="False" w713 {
              tunnel: w700 -> [w731 w767]
              tunnel: w699 -> [w730 _]
              tunnel: w703 -> [w729 w769]
              tunnel: w702 -> [w728 w768]
              tunnel: w698 -> [w724 _]
              tunnel: [w723 w767] -> w712
              tunnel: [w722 w769] -> w711
              tunnel: [w721 w768] -> w710
              tunnel: w695 -> [w717 _]
              frame False {
                n168 = flat-sequence {
                  tunnel: w731 -> [w740]
                  tunnel: w730 -> [w737]
                  tunnel: w729 -> [w739]
                  tunnel: w728 -> [w738]
                  tunnel: [w736] -> w727
                  tunnel: [w735] -> w726
                  tunnel: [w734] -> w725
                  tunnel: w717 -> [w733]
                  tunnel: [w732] -> w716
                  tunnel: w727 -> [w752]
                  tunnel: w726 -> [w751]
                  tunnel: w725 -> [w750]
                  tunnel: w724 -> [w749]
                  tunnel: [w748] -> w720
                  tunnel: [w747] -> w719
                  tunnel: [w746] -> w718
                  tunnel: w716 -> [w745]
                  tunnel: [w764] -> w721
                  tunnel: [w765] -> w722
                  tunnel: [w766] -> w723
                  tunnel: w720 -> [w766]
                  tunnel: w719 -> [w765]
                  tunnel: w718 -> [w764]
                  frame #0 {
                    n169 = Bundle(cluster=w733, "Velocity (units/s)"=0.0) -> (w732:T3)  [unwired: 1 in]
                    n170 = call <userlib>:"Positioner Group Jog Parameters Set.vi"("Group Jog parameters"=w732, "error in (no error)"=w738, "XPS error in (no error)"=w739, "Positioner Name (250 c max)"=w737, "connection ID in"=w740) -> ("error out"=w741:errorcluster, "XPS error out"=w742:errorcluster, "connection ID out"=w743:T5)  [unwired: 4 in]
                    n171 = call <userlib>:"Group Jog Mode Disable.vi"("error in (no error)"=w741, "XPS error in (no error)"=w742, "Group Name (250 c max)"=w737, "connection ID in"=w743) -> ("error out"=w734:errorcluster, "XPS error out"=w735:errorcluster, "connection ID out"=w736:T5)  [unwired: 5 in]
                  }
                  frame #1 {
                    n172 = call <userlib>:"Positioner Group Jog Parameters Set.vi"("Group Jog parameters"=w745, "error in (no error)"=w750, "XPS error in (no error)"=w751, "Positioner Name (250 c max)"=w749, "connection ID in"=w752) -> ("error out"=w755:errorcluster, "XPS error out"=w754:errorcluster, "connection ID out"=w753:T5)  [unwired: 4 in]
                    n173 = call <userlib>:"Group Jog Mode Disable.vi"("error in (no error)"=w755, "XPS error in (no error)"=w754, "Group Name (250 c max)"=w749, "connection ID in"=w753) -> ("error out"=w746:errorcluster, "XPS error out"=w747:errorcluster, "connection ID out"=w748:T5)  [unwired: 5 in]
                  }
                  frame #2 {
                    n174 = property on="Tab Control" class="TabCtl (strict)"() -> ("Pages"=w757:refnum<vi>[])  [unwired: 2 in, 2 out]
                    n175 = Index Array(array=w757, index=1) -> (element=w759:refnum<vi>)
                    n176 = Index Array(array=w757, index=0) -> (element=w761:refnum<vi>)
                    n177 = property on="Tab Control" class="TabCtl (strict)"("Value"=enum32{"JOG MODE", "MOVE MODE"}."MOVE MODE" ("Tab Control")) -> ()  [unwired: 2 in, 2 out]
                    n178 = property class="Page"(reference=w759, "PageEnb"=T4."Page Enabled" ("Page Enabled State")) -> ()  [unwired: 1 in, 2 out]
                    n179 = property class="Page"(reference=w761, "PageEnb"=T4."Page Disabled" ("Page Enabled State")) -> ()  [unwired: 1 in, 2 out]
                  }
                }
              }
              frame True {
                n180 = One Button Dialog(message="Axes are still moving") -> ()  [unwired: 1 in, 1 out]
              }
            }
          }
        }
      }
      event "Axis 1 move absolute": Value Change {
        n181 = event-data() -> ()  [unwired: 1 in, 6 out]
        n182 = case shown="True" "Axis 1 move absolute" {
          tunnel: w779 -> [w782 w794]
          tunnel: w778 -> [_ w793]
          tunnel: w777 -> [w781 w792]
          tunnel: w776 -> [w780 w791]
          tunnel: [w782 w789] -> w775
          tunnel: [w781 w787] -> w774
          tunnel: [w780 w785] -> w773
          tunnel: w772 -> [_ w783]
          frame False {
          }
          frame True {
            n183 = call "Stage group check.vi"("error in (no error)"=w791, "XPS error in (no error)"=w792, "Group Name (250 c max)"=w793, "connection ID in"=w794) -> ("error out"=w786:errorcluster, "XPS error out"=w788:errorcluster, "Stages ready?"=w795:bool, "connection ID out"=w790:T5, "Group Name (250 c max) 2"=w784:string)  [unwired: 3 in]
            n184 = case shown="True" w795 {
              tunnel: w790 -> [w798 w811]
              tunnel: [w798 w802] -> w789
              tunnel: w788 -> [w797 w809]
              tunnel: [w797 w801] -> w787
              tunnel: w786 -> [w796 w808]
              tunnel: [w796 w800] -> w785
              tunnel: w784 -> [_ w810]
              tunnel: w783 -> [_ w807]
              frame False {
                n185 = One Button Dialog(message="Stage 1 is not ready") -> ()  [unwired: 1 in, 1 out]
              }
              frame True {
                n186 = flat-sequence {
                  tunnel: w811 -> [w823]
                  tunnel: w810 -> [w812]
                  tunnel: w809 -> [w822]
                  tunnel: w808 -> [w821]
                  tunnel: w807 -> [w820]
                  tunnel: [w817] -> w806
                  tunnel: [w816] -> w805
                  tunnel: [w815] -> w804
                  tunnel: [w813] -> w803
                  tunnel: w806 -> [w831]
                  tunnel: w805 -> [w830]
                  tunnel: w804 -> [w829]
                  tunnel: w803 -> [w828]
                  tunnel: [w827] -> w802
                  tunnel: [w826] -> w801
                  tunnel: [w825] -> w800
                  frame #0 {
                    n187 = Concatenate Strings(w812, ".Pos" ("string")) -> (w813:string)
                    n188 = local read "Velocity (slow)"() -> (w819:dbl)
                    n189 = Bundle(cluster=w820, "Velocity (units/seconds)"=w819) -> (w818:T2)  [unwired: 3 in]
                    n190 = call <userlib>:"Positioner SGamma Parameters Set.vi"("SGamma Parameters"=w818, "error in (no error)"=w821, "XPS error in (no error)"=w822, "Positioner Name (250 c max)"=w813, "connection ID in"=w823) -> ("error out"=w815:errorcluster, "XPS error out"=w816:errorcluster, "connection ID out"=w817:T5)  [unwired: 4 in]
                  }
                  frame #1 {
                    n191 = local read "Absolute"() -> (w824:dbl)
                    n192 = call <userlib>:"Single Axis Group Move Absolute.vi"("Target Position (units)"=w824, "error in (no error)"=w829, "XPS error in (no error)"=w830, "SingleAxis Group  Name (250 c max)"=w828, "connection ID in"=w831) -> ("error out"=w825:errorcluster, "XPS error out"=w826:errorcluster, "connection ID out"=w827:T5)  [unwired: 4 in]
                  }
                }
              }
            }
          }
        }
      }
      event "Axis 1 move relative": Value Change {
        n193 = event-data() -> ()  [unwired: 1 in, 6 out]
        n194 = case shown="True" "Axis 1 move relative" {
          tunnel: w839 -> [w843 w855]
          tunnel: w836 -> [_ w854]
          tunnel: w838 -> [w842 w853]
          tunnel: w837 -> [w841 w852]
          tunnel: [w843 w850] -> w834
          tunnel: [w842 w848] -> w833
          tunnel: [w841 w846] -> w832
          tunnel: w840 -> [_ w844]
          frame False {
          }
          frame True {
            n195 = call "Stage group check.vi"("error in (no error)"=w852, "XPS error in (no error)"=w853, "Group Name (250 c max)"=w854, "connection ID in"=w855) -> ("error out"=w847:errorcluster, "XPS error out"=w849:errorcluster, "Stages ready?"=w856:bool, "connection ID out"=w851:T5, "Group Name (250 c max) 2"=w845:string)  [unwired: 3 in]
            n196 = case shown="True" w856 {
              tunnel: w851 -> [w859 w872]
              tunnel: [w859 w863] -> w850
              tunnel: w849 -> [w858 w870]
              tunnel: [w858 w862] -> w848
              tunnel: w847 -> [w857 w869]
              tunnel: [w857 w861] -> w846
              tunnel: w845 -> [_ w871]
              tunnel: w844 -> [_ w868]
              frame False {
                n197 = One Button Dialog(message="Stage 1 is not ready") -> ()  [unwired: 1 in, 1 out]
              }
              frame True {
                n198 = flat-sequence {
                  tunnel: w872 -> [w884]
                  tunnel: w871 -> [w874]
                  tunnel: w870 -> [w883]
                  tunnel: w869 -> [w882]
                  tunnel: w868 -> [w881]
                  tunnel: [w878] -> w867
                  tunnel: [w877] -> w866
                  tunnel: [w876] -> w865
                  tunnel: [w873] -> w864
                  tunnel: w867 -> [w892]
                  tunnel: w866 -> [w891]
                  tunnel: w865 -> [w890]
                  tunnel: w864 -> [w889]
                  tunnel: [w888] -> w863
                  tunnel: [w887] -> w862
                  tunnel: [w886] -> w861
                  frame #0 {
                    n199 = Concatenate Strings(w874, ".Pos" ("string")) -> (w873:string)
                    n200 = local read "Velocity (slow)"() -> (w880:dbl)
                    n201 = Bundle(cluster=w881, "Velocity (units/seconds)"=w880) -> (w879:T2)  [unwired: 3 in]
                    n202 = call <userlib>:"Positioner SGamma Parameters Set.vi"("SGamma Parameters"=w879, "error in (no error)"=w882, "XPS error in (no error)"=w883, "Positioner Name (250 c max)"=w873, "connection ID in"=w884) -> ("error out"=w876:errorcluster, "XPS error out"=w877:errorcluster, "connection ID out"=w878:T5)  [unwired: 4 in]
                  }
                  frame #1 {
                    n203 = local read "Relative"() -> (w885:dbl)
                    n204 = call <userlib>:"Single Axis Group Move Relative.vi"("Target Displacement (units)"=w885, "error in (no error)"=w890, "XPS error in (no error)"=w891, "SingleAxis Group  Name (250 c max)"=w889, "connection ID in"=w892) -> ("error out"=w886:errorcluster, "XPS error out"=w887:errorcluster, "connection ID out"=w888:T5)  [unwired: 4 in]
                  }
                }
              }
            }
          }
        }
      }
      event "Axis 2 move relative": Value Change {
        n205 = event-data() -> ()  [unwired: 1 in, 6 out]
        n206 = case shown="True" "Axis 2 move relative" {
          tunnel: w900 -> [w904 w916]
          tunnel: w898 -> [_ w915]
          tunnel: w899 -> [w903 w914]
          tunnel: w897 -> [w902 w913]
          tunnel: [w904 w911] -> w895
          tunnel: [w903 w909] -> w894
          tunnel: [w902 w907] -> w893
          tunnel: w901 -> [_ w905]
          frame False {
          }
          frame True {
            n207 = call "Stage group check.vi"("error in (no error)"=w913, "XPS error in (no error)"=w914, "Group Name (250 c max)"=w915, "connection ID in"=w916) -> ("error out"=w908:errorcluster, "XPS error out"=w910:errorcluster, "Stages ready?"=w917:bool, "connection ID out"=w912:T5, "Group Name (250 c max) 2"=w906:string)  [unwired: 3 in]
            n208 = case shown="True" w917 {
              tunnel: w912 -> [w920 w933]
              tunnel: [w920 w924] -> w911
              tunnel: w910 -> [w919 w931]
              tunnel: [w919 w923] -> w909
              tunnel: w908 -> [w918 w930]
              tunnel: [w918 w922] -> w907
              tunnel: w906 -> [_ w932]
              tunnel: w905 -> [_ w929]
              frame False {
                n209 = One Button Dialog(message="Stage 1 is not ready") -> ()  [unwired: 1 in, 1 out]
              }
              frame True {
                n210 = flat-sequence {
                  tunnel: w933 -> [w945]
                  tunnel: w932 -> [w934]
                  tunnel: w931 -> [w944]
                  tunnel: w930 -> [w943]
                  tunnel: w929 -> [w942]
                  tunnel: [w940] -> w928
                  tunnel: [w939] -> w927
                  tunnel: [w938] -> w926
                  tunnel: [w935] -> w925
                  tunnel: w928 -> [w953]
                  tunnel: w927 -> [w952]
                  tunnel: w926 -> [w951]
                  tunnel: w925 -> [w950]
                  tunnel: [w949] -> w924
                  tunnel: [w948] -> w923
                  tunnel: [w947] -> w922
                  frame #0 {
                    n211 = Concatenate Strings(w934, ".Pos" ("string")) -> (w935:string)
                    n212 = local read "Axis 2 Velocity (slow)\nmm/s"() -> (w937:dbl)
                    n213 = Bundle(cluster=w942, "Velocity (units/seconds)"=w937) -> (w941:T2)  [unwired: 3 in]
                    n214 = call <userlib>:"Positioner SGamma Parameters Set.vi"("SGamma Parameters"=w941, "error in (no error)"=w943, "XPS error in (no error)"=w944, "Positioner Name (250 c max)"=w935, "connection ID in"=w945) -> ("error out"=w938:errorcluster, "XPS error out"=w939:errorcluster, "connection ID out"=w940:T5)  [unwired: 4 in]
                  }
                  frame #1 {
                    n215 = local read "Relative Axis 2"() -> (w946:dbl)
                    n216 = call <userlib>:"Single Axis Group Move Relative.vi"("Target Displacement (units)"=w946, "error in (no error)"=w951, "XPS error in (no error)"=w952, "SingleAxis Group  Name (250 c max)"=w950, "connection ID in"=w953) -> ("error out"=w947:errorcluster, "XPS error out"=w948:errorcluster, "connection ID out"=w949:T5)  [unwired: 4 in]
                  }
                }
              }
            }
          }
        }
      }
      event "Axis 2 move absolute": Value Change {
        n217 = event-data() -> ()  [unwired: 1 in, 6 out]
        n218 = case shown="True" "Axis 2 move absolute" {
          tunnel: w962 -> [w965 w977]
          tunnel: w959 -> [_ w976]
          tunnel: w961 -> [w964 w975]
          tunnel: w960 -> [w963 w974]
          tunnel: [w965 w972] -> w956
          tunnel: [w964 w970] -> w955
          tunnel: [w963 w968] -> w954
          tunnel: w958 -> [_ w966]
          frame False {
          }
          frame True {
            n219 = call "Stage group check.vi"("error in (no error)"=w974, "XPS error in (no error)"=w975, "Group Name (250 c max)"=w976, "connection ID in"=w977) -> ("error out"=w969:errorcluster, "XPS error out"=w971:errorcluster, "Stages ready?"=w978:bool, "connection ID out"=w973:T5, "Group Name (250 c max) 2"=w967:string)  [unwired: 3 in]
            n220 = case shown="True" w978 {
              tunnel: w973 -> [w981 w994]
              tunnel: [w981 w985] -> w972
              tunnel: w971 -> [w980 w992]
              tunnel: [w980 w984] -> w970
              tunnel: w969 -> [w979 w991]
              tunnel: [w979 w983] -> w968
              tunnel: w967 -> [_ w993]
              tunnel: w966 -> [_ w990]
              frame False {
                n221 = One Button Dialog(message="Stage 1 is not ready") -> ()  [unwired: 1 in, 1 out]
              }
              frame True {
                n222 = flat-sequence {
                  tunnel: w994 -> [w1006]
                  tunnel: w993 -> [w995]
                  tunnel: w992 -> [w1005]
                  tunnel: w991 -> [w1004]
                  tunnel: w990 -> [w1003]
                  tunnel: [w1001] -> w989
                  tunnel: [w1000] -> w988
                  tunnel: [w999] -> w987
                  tunnel: [w996] -> w986
                  tunnel: w989 -> [w1014]
                  tunnel: w988 -> [w1013]
                  tunnel: w987 -> [w1012]
                  tunnel: w986 -> [w1011]
                  tunnel: [w1010] -> w985
                  tunnel: [w1009] -> w984
                  tunnel: [w1008] -> w983
                  frame #0 {
                    n223 = Concatenate Strings(w995, ".Pos" ("string")) -> (w996:string)
                    n224 = local read "Axis 2 Velocity (slow)\nmm/s"() -> (w998:dbl)
                    n225 = Bundle(cluster=w1003, "Velocity (units/seconds)"=w998) -> (w1002:T2)  [unwired: 3 in]
                    n226 = call <userlib>:"Positioner SGamma Parameters Set.vi"("SGamma Parameters"=w1002, "error in (no error)"=w1004, "XPS error in (no error)"=w1005, "Positioner Name (250 c max)"=w996, "connection ID in"=w1006) -> ("error out"=w999:errorcluster, "XPS error out"=w1000:errorcluster, "connection ID out"=w1001:T5)  [unwired: 4 in]
                  }
                  frame #1 {
                    n227 = local read "Absolute Axis 2"() -> (w1007:dbl)
                    n228 = call <userlib>:"Single Axis Group Move Absolute.vi"("Target Position (units)"=w1007, "error in (no error)"=w1012, "XPS error in (no error)"=w1013, "SingleAxis Group  Name (250 c max)"=w1011, "connection ID in"=w1014) -> ("error out"=w1008:errorcluster, "XPS error out"=w1009:errorcluster, "connection ID out"=w1010:T5)  [unwired: 4 in]
                  }
                }
              }
            }
          }
        }
      }
    }
    n229 = call <vilib>:"General Error Handler.vi"("[error source] (\" \")"="Standard" ("[error source] (\" \")"), "error in (no error)"=w170) -> ("error out"=w160:errorcluster)  [unwired: 9 in, 4 out]
    n230 = call <vilib>:"General Error Handler.vi"("[error source] (\" \")"="XPS" ("[error source] (\" \")"), "error in (no error)"=w171) -> ("error out"=w168:errorcluster)  [unwired: 9 in, 4 out]
    n231 = call <vilib>:"Clear Errors.vi"("error in (no error)"=w160, "specific error code to clear (0: all)"=42 ("y")) -> ("error out"=w159:errorcluster)  [unwired: 4 in, 1 out]
    n232 = call <vilib>:"Clear Errors.vi"("error in (no error)"=w168, "specific error code to clear (0: all)"=42 ("y")) -> ("error out"=w162:errorcluster)  [unwired: 4 in, 1 out]
  }
  n233 = property on="Axis 2 Velocity (fast)\nmm/s" class="DigNum (strict)"("Maximum"=w7) -> ()  [unwired: 2 in, 2 out]
  n234 = property on="Axis 2 Velocity (slow)\nmm/s" class="DigNum (strict)"("Maximum"=w7) -> ()  [unwired: 2 in, 2 out]
  n235 = property on="Absolute Axis 2" class="DigNum (strict)"("Data Range"=w4) -> ()  [unwired: 2 in, 2 out]
  n236 = property on="Relative Axis 2" class="DigNum (strict)"("Data Range"=w3) -> ()  [unwired: 2 in, 2 out]
  n237 = property on="Absolute" class="DigNum (strict)"("Data Range"=w2) -> ()  [unwired: 2 in, 2 out]
  n238 = property on="Relative" class="DigNum (strict)"("Data Range"=w1) -> ()  [unwired: 2 in, 2 out]
  n239 = property on="Velocity (slow)" class="DigNum (strict)"("Maximum"=w6) -> ()  [unwired: 2 in, 2 out]
  n240 = property on="Velocity (fast)" class="DigNum (strict)"("Maximum"=w6) -> ()  [unwired: 2 in, 2 out]
